vi "reboot camera.vi"(8 "error in (no error)":errorcluster, 11 "Real Camera in":refnum<class "iKon-L.lvclass">) -> (0 "error out":errorcluster, 3 "Real Camera out":refnum<class "iKon-L.lvclass">)   [LabVIEW 2018, in "iKon-L.lvclass"]
uses:
  iKon-L.lvclass
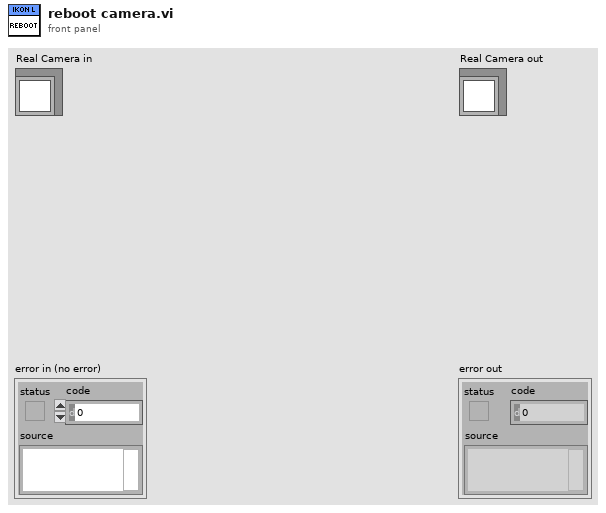
[diagram p1: front panel]
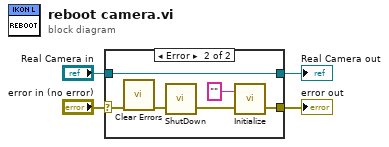
[diagram p0: block diagram]
diagram:
  n1 = case shown="Error" "error in (no error)" {
    selector: "error in (no error)" -> [w5 w11]
    tunnel: [w5 w7] -> w3
    tunnel: [w6 w12] -> w1
    tunnel: "Real Camera in" -> [w6 w12]
    frame No Error {
    }
    frame Error {
      n2 = call <vilib>:"Clear Errors.vi"("error in (no error)"=w11) -> ("error out"=w10:errorcluster)  [unwired: 5 in, 1 out]
      n3 = call <userlib>:"ShutDown.vi"("error in (no error)"=w10) -> ("error out"=w9:errorcluster)  [unwired: 1 in, 1 out]
      n4 = call <userlib>:"Initialize.vi"("error in (no error)"=w9, "directory (\"\")"="" ("directory (\"\")")) -> ("error out"=w7:errorcluster)  [unwired: 1 out]
    }
  }
  "error out" <- w3
  "Real Camera out" <- w1
